vi "Get_Instrument_Instance.vi"(8 "error in (no error)":errorcluster, 10 "session reservation":refnum<class "Session Reservation.lvclass">) -> (0 "error out":errorcluster, 2 "Instruments":refnum<class "Abstract_Instrument.lvclass">[](array[class]))   [LabVIEW 2020, in "Abstract_Instrument.lvlib" / "Abstract_Instrument.lvclass"]
doc: "The API helps in getting the instrument instances that are connnected to the pins given for <b>Reserve Sessions</b> API."
uses:
  Abstract_Instrument.lvclass
  <vilib>/MeasurementLink/MeasurementLink Session Management V1/Session Reservation/Session Reservation.lvclass
  <vilib>/MeasurementLink/MeasurementLink Session Management V1/Session Reservation/Session Reservation.lvclass/Session Reservation.ctl
  <vilib>/MeasurementLink/MeasurementLink Session Management V1/Session Reservation/Get Session Info - NSess .vi
  <vilib>/MeasurementLink/MeasurementLink Session Management V1/Session Reservation/Merge Invalid DVR Error.vi
  <vilib>/MeasurementLink/MeasurementLink Session Management V1/Session Reservation/Is DVR Valid.vi
  <vilib>/MeasurementLink/MeasurementLink Measurement Server/Helpers/Error Strings Global Internal.vi
  <vilib>/Utility/error.llb/Error Cluster From Error Code.vi
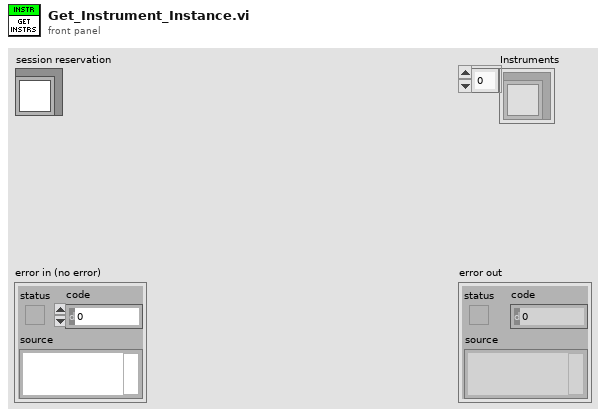
[diagram p1: front panel]
types:
  T1 = typedef "MeasurementLink Session Management Client.lvlib/ni_measurementlink_sessionmanagement_v1_SessionInformation.ctl" = cluster{"session":T2, "resource_name":string, "channel_list":string, "instrument_type_id":string, "session_exists":bool, "channel_mappings":T3[]}
  T2 = typedef "MeasurementLink Session Management Client.lvlib/nidevice_grpc_Session.ctl" = cluster{"name":string}
  T3 = typedef "MeasurementLink Session Management Client.lvlib/ni_measurementlink_sessionmanagement_v1_ChannelMapping.ctl" = cluster{"pin_or_relay_name":string, "site":i32, "channel":string, "multiplexer_resource_name":string, "multiplexer_route":string}
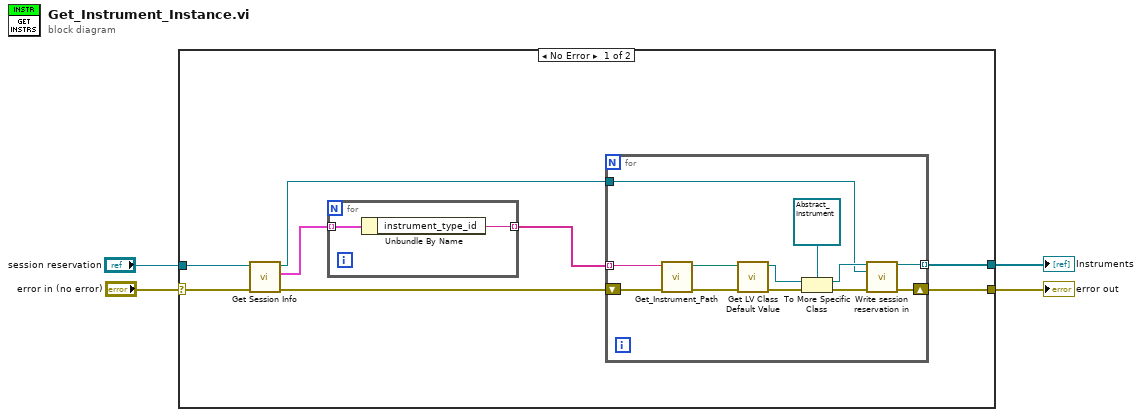
[diagram p0: block diagram]
diagram:
  n1 = case shown="No Error" "error in (no error)" {
    selector: "error in (no error)" -> [w12 w27]
    tunnel: [w10 w27] -> w3
    tunnel: [w7 _] -> w2
    tunnel: "session reservation" -> [w5 _]
    frame No Error {
      n2 = call-poly <vilib>:"Get Session Info.vi"("error in"=w12, "session reservation in"=w5) -> ("error out"=w9:errorcluster, "sessions info"=w11:T1[], "session reservation out"=w6:refnum<class "Session Reservation.lvclass">)  [unwired: 7 in]
      n3 = for {
        tunnel: [w26] -> w8 mode=indexing
        tunnel: w11 -> [w25] mode=indexing
        n4 = Unbundle By Name(w25) -> ("instrument_type_id"=w26:string)
      }
      n5 = for {
        shift-right: [w19] -> w10
        shift-left: w9 -> [w21]
        tunnel: w8 -> [w15] mode=indexing
        tunnel: [w17] -> w7 mode=indexing
        tunnel: w6 -> [w16]
        n6 = call "Get_Instrument_Path.vi"("error in (no error)"=w21, "instrument_type_id"=w15) -> ("error out"=w22:errorcluster, "InstrumentClassPath"=w14:path)  [unwired: 8 in]
        n7 = call <vilib>:"Get LV Class Default Value.vi"("error in (no error)"=w22, "class path"=w14) -> ("error out"=w24:errorcluster, "object"=w23:refnum<class>)  [unwired: 8 in]
        n8 = To More Specific Class(target class=refnum<class "Abstract_Instrument.lvclass"> refnum ("Abstract_Instrument in"), reference=w23, error in=w24) -> (specific class reference=w18:refnum<class "Abstract_Instrument.lvclass">, error out=w20:errorcluster)
        n9 = call-dynamic "Write session reservation in.vi"("AbstractDMM in"=w18, "MeasurementLink Session Management V1.lvlib:Session Reservation.lvclass"=w16, "error in (no error)"=w20) -> ("AbstractDMM out"=w17:refnum<class "Abstract_Instrument.lvclass">, "error out"=w19:errorcluster)  [unwired: 11 in]
      }
    }
    frame Error {
    }
  }
  "error out" <- w3
  "Instruments" <- w2
